vi "Init.vi"(7 "I2C #":T1=-1, 8 "error in (no error)":errorcluster, 10 "Session In":refnum<class "Session.lvclass">) -> (0 "error out":errorcluster, 3 "Grove I2C LCD out":refnum<class "Grove I2C LCD.lvclass">)   [LabVIEW 2020, in "CTI-Peripheral.lvlib" / "Grove I2C LCD.lvclass"]
uses:
  Grove I2C LCD.lvclass
  CTI/I2C Number.ctl
  CTI/Session/Session.lvclass
  HD44780 LCD/Display Function.ctl
  Character LCD/Bus Mode.ctl
  Character LCD/Lines.ctl
  Character LCD/Glyph Size.ctl
  HD44780 LCD/Display Mode.ctl
  Character LCD/Entry Shift.ctl
  Character LCD/Glyph Entry.ctl
  HD44780 LCD/Display Control.ctl
  HD44780 LCD/Command.ctl
  CTI/I2C Address.ctl
  CTI/I2C Connection/I2C Connection.lvclass/I2C Connection.ctl
  Grove I2C LCD.lvclass/Grove I2C LCD.ctl
  9b7d9e7c-47ba-483e-8c4c-ef7aeef1a812.vi
  7e84b810-20cf-4811-a4e1-4dc61167239c.vi
  CTI/I2C Connection/I2C Connection.lvclass
  HD44780 LCD/HD44780 LCD.lvlib
  Character LCD/Char LCD.lvclass
  CTI/CTI.lvlib
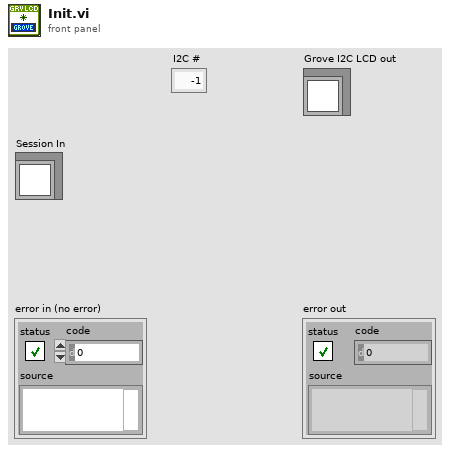
[diagram p1: front panel]
types:
  T1 = typedef "CTI.lvlib/I2C Number.ctl" = i8
  T2 = typedef "CTI.lvlib/I2C Address.ctl" = u8
  T3 = typedef "CTI-Peripheral.lvlib/HD44780 LCD.lvlib/Command.ctl" = enum16{"ClearDisplay", "ReturnHome", "EntryModeSet", "DisplayControl", "CursorShift", "FunctionSet", "SetCGRamAddr", "SetDDRamAddr"}
  T4 = typedef "CTI-Peripheral.lvlib/HD44780 LCD.lvlib/Display Control.ctl" = cluster{"Blink On":bool, "Cursor On":bool, "Display On":bool}
  T5 = typedef "CTI-Peripheral.lvlib/HD44780 LCD.lvlib/Display Mode.ctl" = cluster{"Entry Shift":T6, "Glyph Entry":T7}
  T6 = typedef "CTI-Peripheral.lvlib/Char LCD.lvclass/Entry Shift.ctl" = enum8{"Decrement", "Increment"}
  T7 = typedef "CTI-Peripheral.lvlib/Char LCD.lvclass/Glyph Entry.ctl" = enum8{"Right", "Left"}
  T8 = typedef "CTI-Peripheral.lvlib/HD44780 LCD.lvlib/Display Function.ctl" = cluster{"Bus Mode":T9, "Lines":T10, "Glyph Size":T11}
  T9 = typedef "CTI-Peripheral.lvlib/Char LCD.lvclass/Bus Mode.ctl" = enum8{"4 Bit", "8 Bit"}
  T10 = typedef "CTI-Peripheral.lvlib/Char LCD.lvclass/Lines.ctl" = enum8{"Single", "Multiline"}
  T11 = typedef "CTI-Peripheral.lvlib/Char LCD.lvclass/Glyph Size.ctl" = enum8{"5x8", "5x10"}
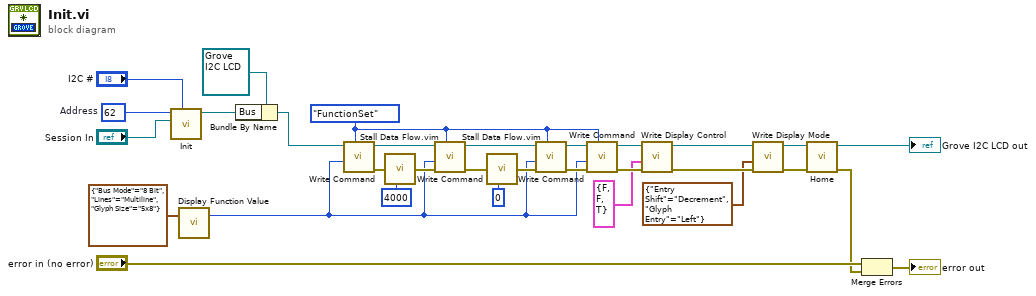
[diagram p0: block diagram]
diagram:
  w28 = T2 62  # Address
  w15 = Command."FunctionSet" ("Command")
  n1 = call "Init.vi"("I2C #"="I2C #", "Session"="Session In", "Address"=w28) -> ("I2C Connection"=w26:refnum<class "I2C Connection.lvclass">)  [unwired: 7 in, 1 out]
  n2 = call "Display Function Value.vi"("Display Function"=T8 {"Bus Mode"=enum."8 Bit", "Lines"=enum."Multiline", "Glyph Size"=enum."5x8"}) -> ("DisplayFunc"=w12:u8)  [unwired: 6 in]
  n3 = Bundle By Name(cluster=refnum<class "Grove I2C LCD.lvclass"> refnum ("Grove I2C LCD in"), "Bus"=w26) -> (w27:refnum<class "Grove I2C LCD.lvclass">)
  n4 = call "Write Command.vi"("Command"=w15, "Value"=w12, "Grove I2C LCD in"=w27) -> ("error out"=w23:errorcluster, "Grove I2C LCD out"=w16:refnum<class "Grove I2C LCD.lvclass">)  [unwired: 7 in]
  n5 = call "Stall Data Flow.vim"("value in"=w23, "milliseconds to wait"=u32 4000) -> ("value out"=w22:errorcluster)  [unwired: 1 out]
  n6 = call "Write Command.vi"("Command"=w15, "error in (no error)"=w22, "Value"=w12, "Grove I2C LCD in"=w16) -> ("error out"=w20:errorcluster, "Grove I2C LCD out"=w17:refnum<class "Grove I2C LCD.lvclass">)  [unwired: 6 in]
  n7 = call "Stall Data Flow.vim"("value in"=w20, "milliseconds to wait"=u32 0) -> ("value out"=w18:errorcluster)  [unwired: 1 out]
  n8 = call "Write Command.vi"("Command"=w15, "error in (no error)"=w18, "Value"=w12, "Grove I2C LCD in"=w17) -> ("error out"=w14:errorcluster, "Grove I2C LCD out"=w13:refnum<class "Grove I2C LCD.lvclass">)  [unwired: 6 in]
  n9 = call "Write Command.vi"("Command"=w15, "error in (no error)"=w14, "Value"=w12, "Grove I2C LCD in"=w13) -> ("error out"=w10:errorcluster, "Grove I2C LCD out"=w11:refnum<class "Grove I2C LCD.lvclass">)  [unwired: 6 in]
  n10 = call "Write Display Control.vi"("error in (no error)"=w10, "Display Control"=T4 {"Blink On"=FALSE, "Cursor On"=FALSE, "Display On"=TRUE}, "Grove I2C LCD in"=w11) -> ("error out"=w8:errorcluster, "Grove I2C LCD out"=w7:refnum<class "Grove I2C LCD.lvclass">)  [unwired: 7 in]
  n11 = call "Write Display Mode.vi"("error in (no error)"=w8, "Display Mode"=T5 {"Entry Shift"=enum."Decrement", "Glyph Entry"=enum."Left"}, "Grove I2C LCD in"=w7) -> ("error out"=w5:errorcluster, "Grove I2C LCD out"=w3:refnum<class "Grove I2C LCD.lvclass">)  [unwired: 7 in]
  n12 = call-dynamic "Home.vi"("error in (no error)"=w5, "Character LCD in"=w3) -> ("error out"=w4:errorcluster, "Character LCD out"=→"Grove I2C LCD out":refnum<class "Grove I2C LCD.lvclass">)  [unwired: 8 in]
  n13 = Merge Errors("error in (no error)", w4) -> (→"error out":errorcluster)
